vi "Control Board - Read.vi"(8 "error in (no error)":errorcluster, 11 "VISA Refnum in":refnum<visa-resource-name>) -> (0 "error out":errorcluster, 1 "Analog Inputs":T1, 2 "Switch Inputs":T2, 3 "VISA Refnum out":refnum<visa-resource-name>)   [LabVIEW 2015]
uses:
  Switch_Input_TypeDef.ctl
  Analog_Input_TypeDef.ctl
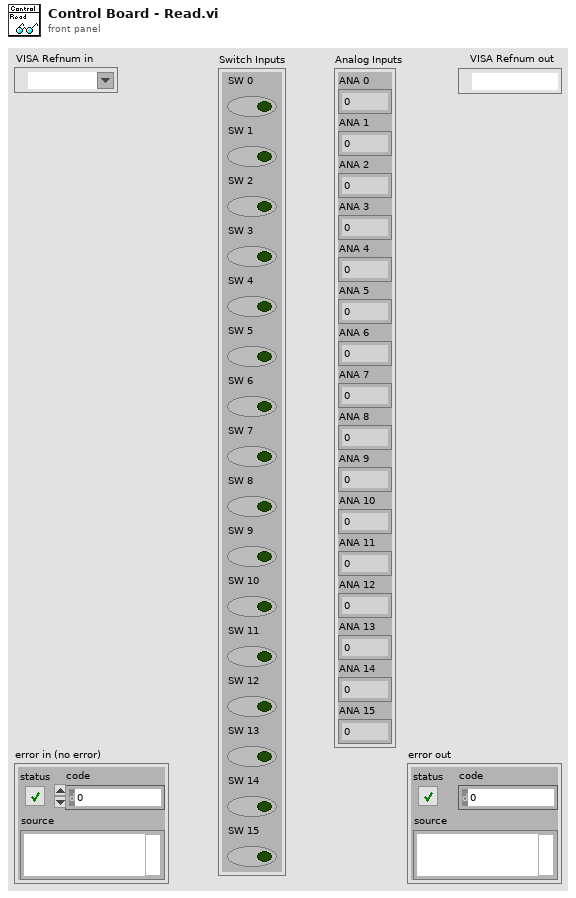
[diagram p1: front panel]
types:
  T1 = typedef "Analog_Input_TypeDef.ctl" = cluster{"ANA 0":u8, "ANA 1":u8, "ANA 2":u8, "ANA 3":u8, "ANA 4":u8, "ANA 5":u8, "ANA 6":u8, "ANA 7":u8, "ANA 8":u8, "ANA 9":u8, "ANA 10":u8, "ANA 11":u8, "ANA 12":u8, "ANA 13":u8, "ANA 14":u8, "ANA 15":u8}
  T2 = typedef "Switch_Input_TypeDef.ctl" = cluster{"SW 0":bool, "SW 1":bool, "SW 2":bool, "SW 3":bool, "SW 4":bool, "SW 5":bool, "SW 6":bool, "SW 7":bool, "SW 8":bool, "SW 9":bool, "SW 10":bool, "SW 11":bool, "SW 12":bool, "SW 13":bool, "SW 14":bool, "SW 15":bool}
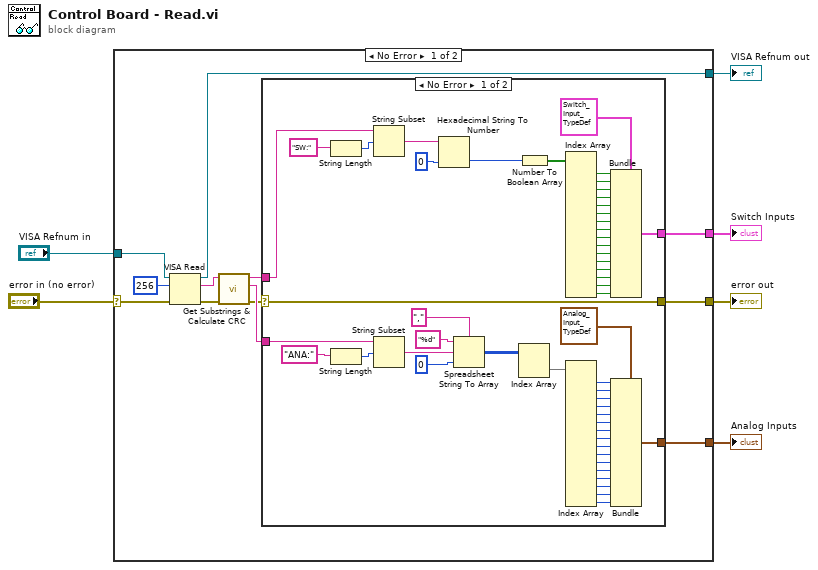
[diagram p0: block diagram]
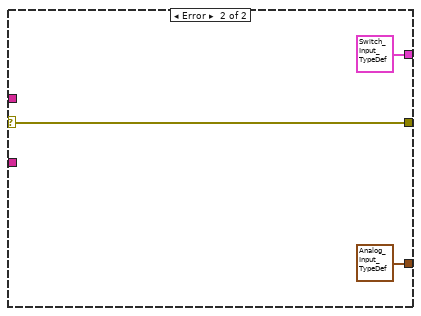
[diagram p2: hidden frame]
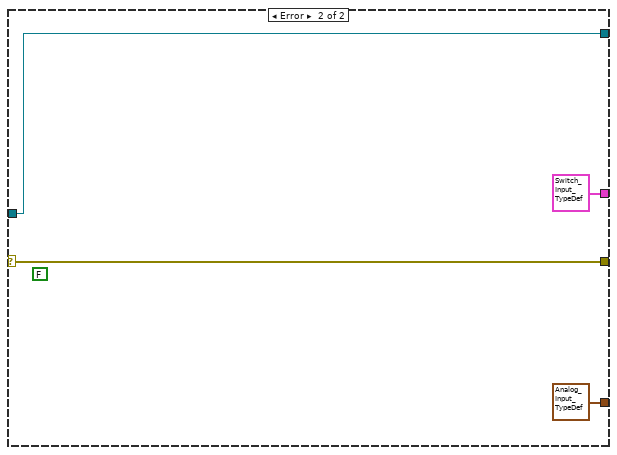
[diagram p3: hidden frame]
diagram:
  n1 = case shown="No Error" "error in (no error)" {
    selector: "error in (no error)" -> [w8 w77]
    tunnel: [w17 w78] -> w6
    tunnel: "VISA Refnum in" -> [w15 w78]
    tunnel: [w13 T2 {"SW 0"=FALSE, "SW 1"=FALSE, "SW 2"=FALSE, "SW 3"=FALSE, "SW 4"=FALSE, "SW 5"=FALSE, "SW 6"=FALSE, "SW 7"=FALSE, "SW 8"=FALSE, "SW 9"=FALSE, "SW 10"=FALSE, "SW 11"=FALSE, "SW 12"=FALSE, "SW 13"=FALSE, "SW 14"=FALSE, "SW 15"=FALSE} ("Switch Inputs")] -> w4
    tunnel: [w11 w77] -> w3
    tunnel: [w10 T1 {"ANA 0"=0, "ANA 1"=0, "ANA 2"=0, "ANA 3"=0, "ANA 4"=0, "ANA 5"=0, "ANA 6"=0, "ANA 7"=0, "ANA 8"=0, "ANA 9"=0, "ANA 10"=0, "ANA 11"=0, "ANA 12"=0, "ANA 13"=0, "ANA 14"=0, "ANA 15"=0} ("Analog Inputs")] -> w2
    frame No Error {
      n2 = VISA Read(VISA resource name=w15, byte count=u32 256, error in (no error)=w8) -> (VISA resource name out=w17:refnum<visa-resource-name>, read buffer=w18:string, error out=w9:errorcluster)  [unwired: 1 out]
      n3 = call "Get Substrings & Calculate CRC.vi"("error in (no error)"=w9, "Data In"=w18) -> ("error out"=w7:errorcluster, "Analogs"=w12:string, "Switches"=w14:string)  [unwired: 7 in]
      n4 = case shown="No Error" w7 {
        selector: w7 -> [w67 w74]
        tunnel: w14 -> [w71 _]
        tunnel: [w70 T2 {"SW 0"=FALSE, "SW 1"=FALSE, "SW 2"=FALSE, "SW 3"=FALSE, "SW 4"=FALSE, "SW 5"=FALSE, "SW 6"=FALSE, "SW 7"=FALSE, "SW 8"=FALSE, "SW 9"=FALSE, "SW 10"=FALSE, "SW 11"=FALSE, "SW 12"=FALSE, "SW 13"=FALSE, "SW 14"=FALSE, "SW 15"=FALSE} ("Switch Inputs")] -> w13
        tunnel: w12 -> [w69 _]
        tunnel: [w67 w74] -> w11
        tunnel: [w68 T1 {"ANA 0"=0, "ANA 1"=0, "ANA 2"=0, "ANA 3"=0, "ANA 4"=0, "ANA 5"=0, "ANA 6"=0, "ANA 7"=0, "ANA 8"=0, "ANA 9"=0, "ANA 10"=0, "ANA 11"=0, "ANA 12"=0, "ANA 13"=0, "ANA 14"=0, "ANA 15"=0} ("Analog Inputs")] -> w10
        frame No Error {
          n5 = String Length(string="SW:") -> (length=w65:i32)
          n6 = String Length(string="ANA:") -> (length=w30:i32)
          n7 = String Subset(string=w71, offset (0)=w65) -> (substring=w22:string)  [unwired: 1 in]
          n8 = String Subset(string=w69, offset (0)=w30) -> (substring=w27:string)  [unwired: 1 in]
          n9 = Hexadecimal String To Number(string=w22, default (0uL)=u16 0 ("default (0 U32)")) -> (number=w20:u16)  [unwired: 1 in, 1 out]
          n10 = Spreadsheet String To Array(delimiter (Tab)=",", format string="%d", spreadsheet string=w27, array type (2D Dbl)=u8 0) -> (array=w26:u8[][])
          n11 = Index Array(array=w26) -> (element=w25:u8[])  [unwired: 2 in]
          n12 = Number To Boolean Array(number=w20) -> (Boolean array=w19:bool[])
          n13 = Index Array(array=w19) -> (element #1=w63:bool, element #2=w62:bool, element #3=w48:bool, element #4=w49:bool, element #5=w50:bool, element #6=w51:bool, element #7=w52:bool, element #8=w53:bool, element #9=w54:bool, element #10=w55:bool, element #11=w56:bool, element #12=w57:bool, element #13=w58:bool, element #14=w59:bool, element #15=w60:bool, element #16=w61:bool)  [unwired: 16 in]
          n14 = Index Array(array=w25) -> (element #1=w32:u8, element #2=w33:u8, element #3=w47:u8, element #4=w46:u8, element #5=w45:u8, element #6=w44:u8, element #7=w43:u8, element #8=w42:u8, element #9=w41:u8, element #10=w40:u8, element #11=w39:u8, element #12=w38:u8, element #13=w37:u8, element #14=w36:u8, element #15=w35:u8, element #16=w34:u8)  [unwired: 16 in]
          n15 = Bundle(cluster=T2 {"SW 0"=FALSE, "SW 1"=FALSE, "SW 2"=FALSE, "SW 3"=FALSE, "SW 4"=FALSE, "SW 5"=FALSE, "SW 6"=FALSE, "SW 7"=FALSE, "SW 8"=FALSE, "SW 9"=FALSE, "SW 10"=FALSE, "SW 11"=FALSE, "SW 12"=FALSE, "SW 13"=FALSE, "SW 14"=FALSE, "SW 15"=FALSE} ("Switch Inputs"), "SW 0"=w63, "SW 1"=w62, "SW 2"=w48, "SW 3"=w49, "SW 4"=w50, "SW 5"=w51, "SW 6"=w52, "SW 7"=w53, "SW 8"=w54, "SW 9"=w55, "SW 10"=w56, "SW 11"=w57, "SW 12"=w58, "SW 13"=w59, "SW 14"=w60, "SW 15"=w61) -> (w70:T2)
          n16 = Bundle(cluster=T1 {"ANA 0"=0, "ANA 1"=0, "ANA 2"=0, "ANA 3"=0, "ANA 4"=0, "ANA 5"=0, "ANA 6"=0, "ANA 7"=0, "ANA 8"=0, "ANA 9"=0, "ANA 10"=0, "ANA 11"=0, "ANA 12"=0, "ANA 13"=0, "ANA 14"=0, "ANA 15"=0} ("Analog Inputs"), "ANA 0"=w32, "ANA 1"=w33, "ANA 2"=w47, "ANA 3"=w46, "ANA 4"=w45, "ANA 5"=w44, "ANA 6"=w43, "ANA 7"=w42, "ANA 8"=w41, "ANA 9"=w40, "ANA 10"=w39, "ANA 11"=w38, "ANA 12"=w37, "ANA 13"=w36, "ANA 14"=w35, "ANA 15"=w34) -> (w68:T1)
        }
        frame Error {
        }
      }
    }
    frame Error {
      (unwired) FALSE
    }
  }
  "error out" <- w3
  "VISA Refnum out" <- w6
  "Switch Inputs" <- w4
  "Analog Inputs" <- w2
